vi "梦幻城堡C1~3通信.vi"() -> ()   [LabVIEW 2016, in "环境动力监测库.lvlib" / "UPS库.lvlib"]
uses:
  <vilib>/Instr/_visa.llb/VISA Configure Serial Port (Instr).vi
panel:
  out "Status":T1
  in  "open":bool
  in  "close":bool
  out "通信指示":bool
  in  "关机":bool
  in  "状态查询":bool
  out "读取缓冲区":string
  # "输入电压"
  # "输入故障电压"
  # "输出电压"
  # "输出电流百分比"
  # "输入频率"
  # "电池电压"
  # "UPS温度"
  # "UPS状态"
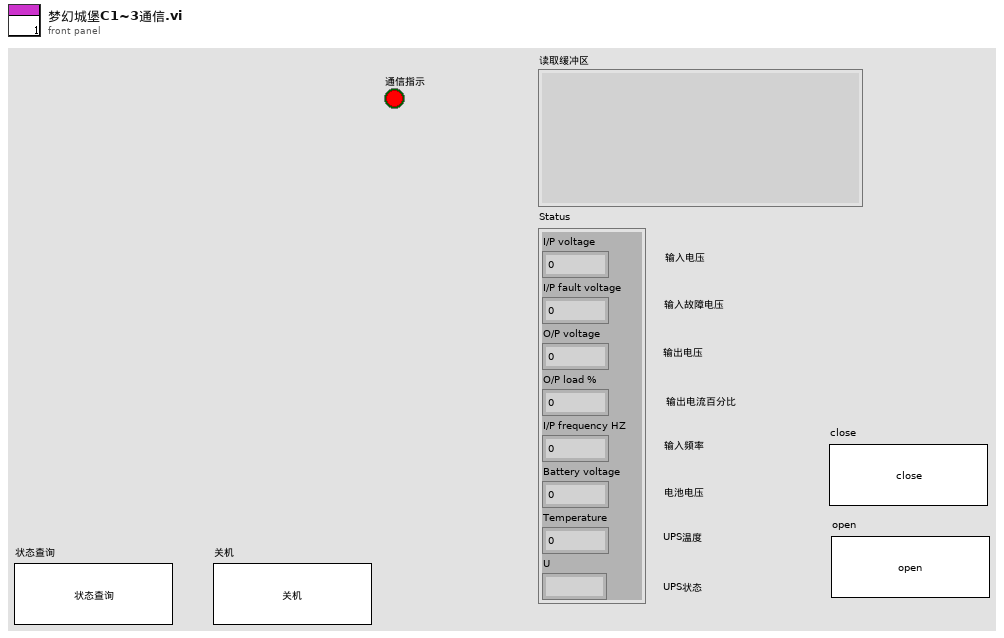
[diagram p1: front panel]
types:
  T1 = cluster{"I/P voltage":dbl, "I/P fault voltage":dbl, "O/P voltage":dbl, "O/P load %":dbl, "I/P frequency HZ":dbl, "Battery voltage":dbl, "Temperature":dbl, "U":string}
  T2 = cluster{"枚举":enum16{"open", "read", "write", "close"}, "写入缓冲区":string}
  T3 = typedef "环境动力监测库.lvlib/UPS库.lvlib/UPS型号.ctl" = enum16{"山特UPSC1~3", "山特UPSC6~20", "华为UPS2000-G-(1-3KVA)", "Kstar"}
  T4 = cluster{"VISA resource name":refnum<visa-resource-name>, "Serial Config":cluster{"baud rate (9600)":u32, "stop bits (10: 1 bit)":u16, "parity (0:none)":enum16{"None", "Odd", "Even", "Mark", "Space"}, "data bits (8)":u16, "timeout (10sec)":u32}, "型号选择":T3, "HW-UPS-2000 MB session":refnum<class "MB_Master.lvclass">, "连接方式":enum16{"串口", "TCP"}, "IP":string, "Port":string, "低电量报警阈值":u16, "功能启用":bool}
  T5 = cluster{"baud rate (9600)":u32, "stop bits (10: 1 bit)":u16, "parity (0:none)":enum16{"None", "Odd", "Even", "Mark", "Space"}, "data bits (8)":u16, "timeout (10sec)":u32}
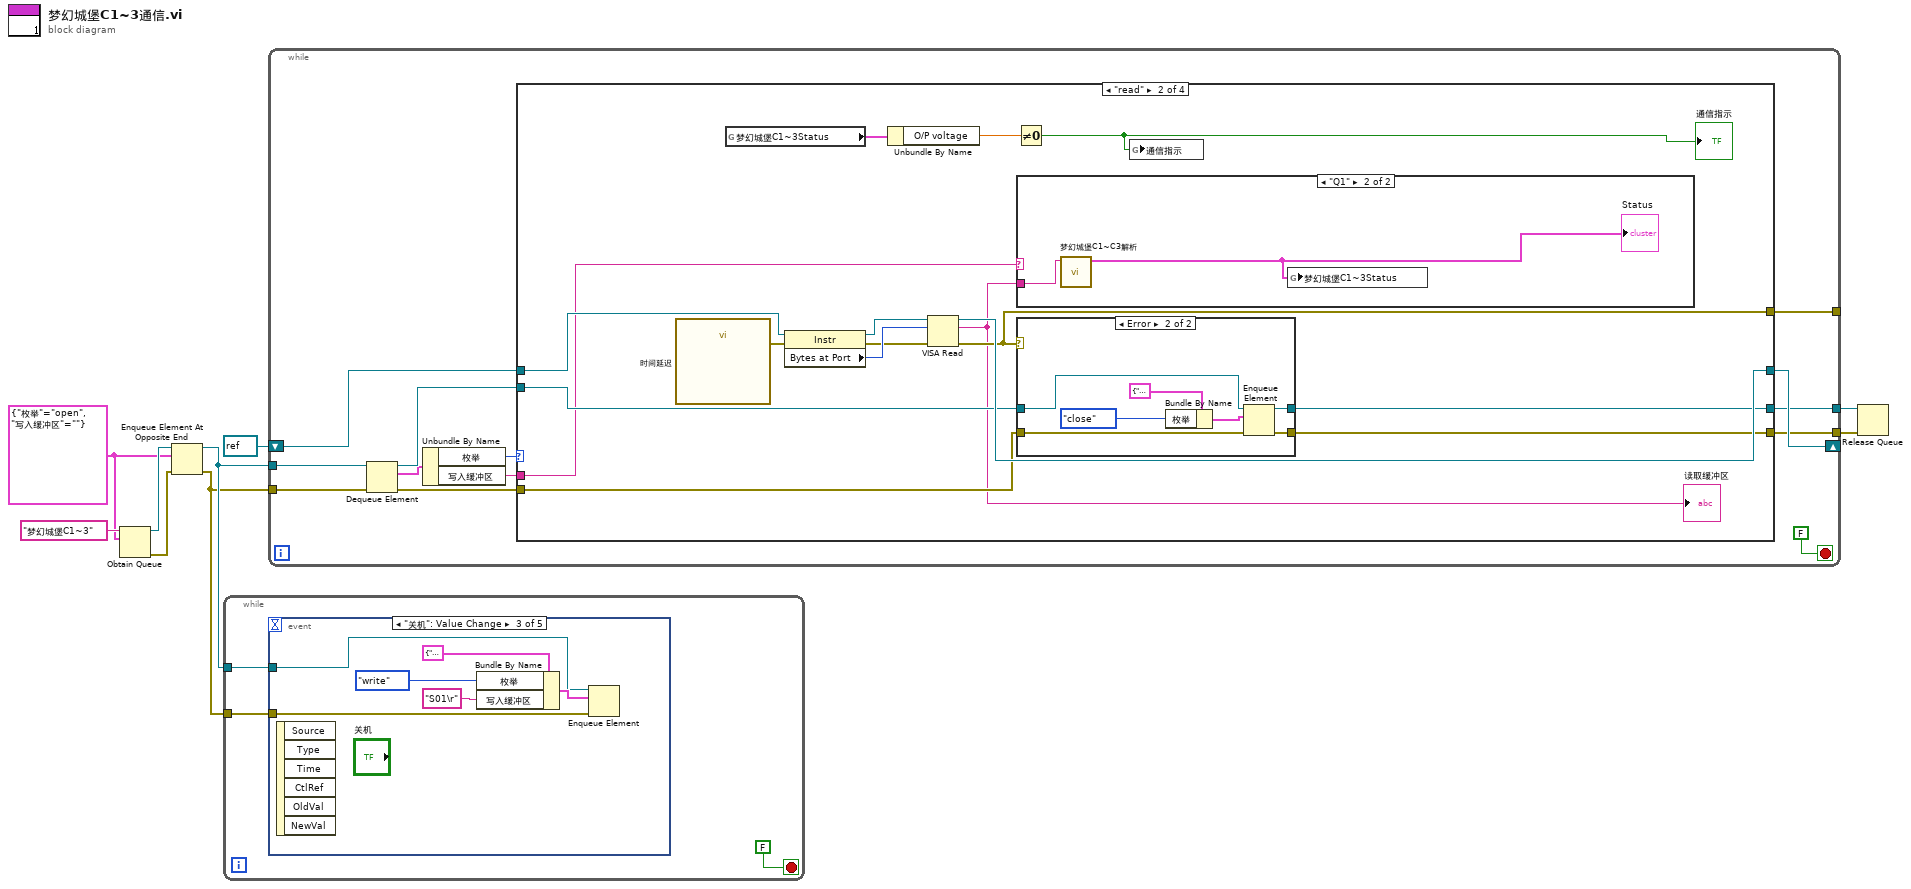
[diagram p0: block diagram]
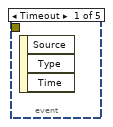
[diagram p2: hidden frame]
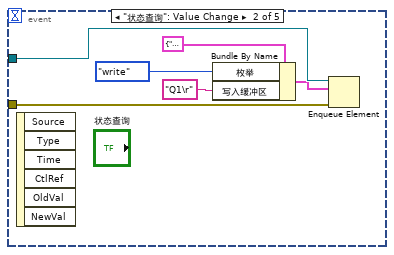
[diagram p3: hidden frame]
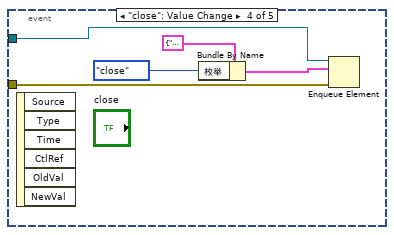
[diagram p4: hidden frame]
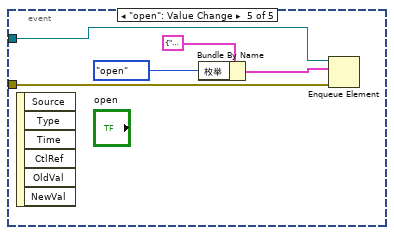
[diagram p5: hidden frame]
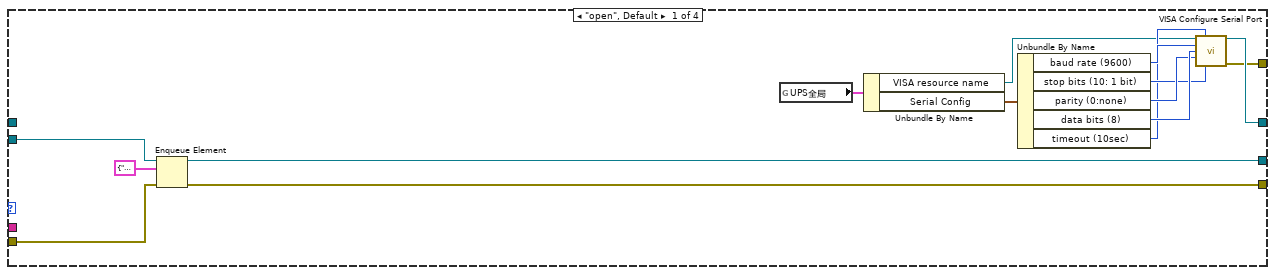
[diagram p6: hidden frame]
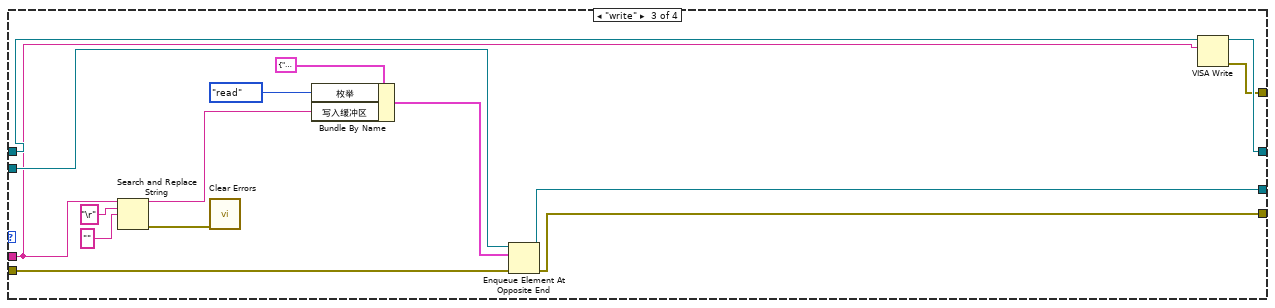
[diagram p9: hidden frame]
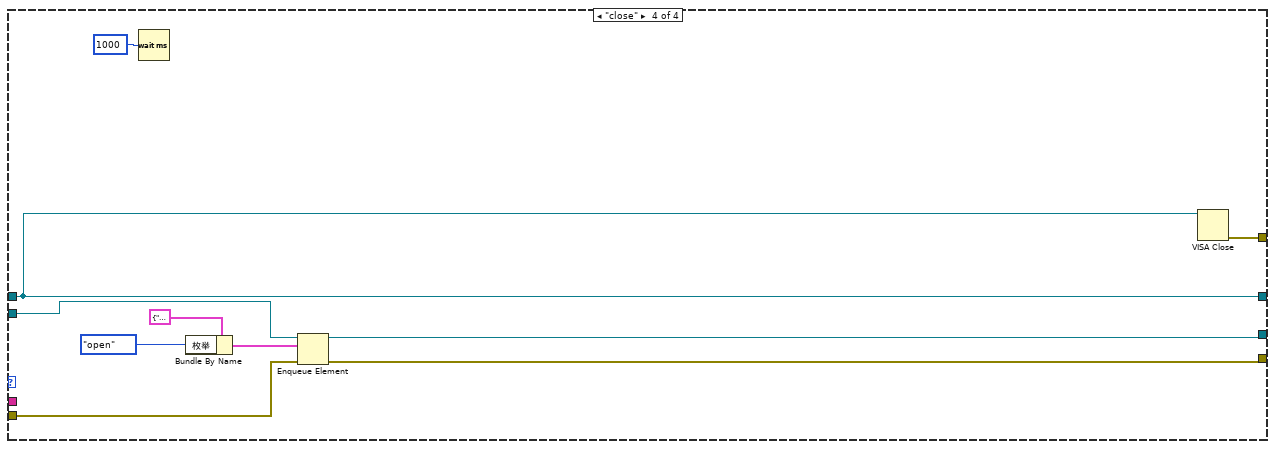
[diagram p10: hidden frame]
diagram:
  w3 = T2 {"枚举"=enum."open", "写入缓冲区"=""}
  n1 = Obtain Queue(name (unnamed)="梦幻城堡C1~3" ("名称（未命名）"), element data type=w3) -> (queue out=w8:refnum<queue>, error out=w7:errorcluster)  [unwired: 3 in, 1 out]
  n2 = Enqueue Element At Opposite End(queue=w8, element=w3, error in (no error)=w7) -> (queue out=w6:refnum<queue>, error out=w5:errorcluster)  [unwired: 1 in, 1 out]
  n3 = while {
    tunnel: w6 -> [w11]
    tunnel: w5 -> [w10]
    stop <- FALSE stop-if-true
    n4 = event shown="[2] \"关机\": Value Change" {
      selector: _ -> [_ _ _ _ _]
      dyn-events: _ -> [_ _ _ _ _]
      timeout: _ -> [_ _ _ _ _]
      tunnel: w11 -> [_ w17 w21 w29 w34]
      tunnel: w10 -> [_ w13 w20 w28 w33]
      event Timeout {
        n5 = event-data() -> ()  [unwired: 1 in, 3 out]
      }
      event "状态查询": Value Change {
        n6 = event-data() -> ()  [unwired: 1 in, 6 out]
        n7 = Bundle By Name(cluster=T2 {"枚举"=enum."open", "写入缓冲区"=""}, "枚举"=enum16{"open", "read", "write", "close"}."write" ("元素"), "写入缓冲区"="Q1\r") -> (w16:T2)
        n8 = Enqueue Element(queue=w17, element=w16, error in (no error)=w13) -> ()  [unwired: 1 in, 3 out]
      }
      event "关机": Value Change {
        n9 = event-data() -> ()  [unwired: 1 in, 6 out]
        n10 = Bundle By Name(cluster=T2 {"枚举"=enum."open", "写入缓冲区"=""}, "枚举"=enum16{"open", "read", "write", "close"}."write" ("元素"), "写入缓冲区"="S01\r") -> (w23:T2)
        n11 = Enqueue Element(queue=w21, element=w23, error in (no error)=w20) -> ()  [unwired: 1 in, 3 out]
      }
      event "close": Value Change {
        n12 = event-data() -> ()  [unwired: 1 in, 6 out]
        n13 = Bundle By Name(cluster=T2 {"枚举"=enum."open", "写入缓冲区"=""}, "枚举"=enum16{"open", "read", "write", "close"}."close") -> (w25:T2)
        n14 = Enqueue Element(queue=w29, element=w25, error in (no error)=w28) -> ()  [unwired: 1 in, 3 out]
      }
      event "open": Value Change {
        n15 = event-data() -> ()  [unwired: 1 in, 6 out]
        n16 = Bundle By Name(cluster=T2 {"枚举"=enum."open", "写入缓冲区"=""}, "枚举"=enum16{"open", "read", "write", "close"}."open") -> (w30:T2)
        n17 = Enqueue Element(queue=w34, element=w30, error in (no error)=w33) -> ()  [unwired: 1 in, 3 out]
      }
    }
  }
  n18 = while {
    shift-right: [w47] -> _
    shift-left: refnum<visa-resource-name> refnum ("VISA resource name out") -> [w46]
    tunnel: [w45] -> _
    tunnel: w6 -> [w43]
    tunnel: w5 -> [w42]
    tunnel: [w38] -> w1
    tunnel: [w39] -> w2
    stop <- FALSE stop-if-true
    n19 = Dequeue Element(queue=w43, error in (no error)=w42) -> (queue out=w41:refnum<queue>, element=w37:T2, error out=w40:errorcluster)  [unwired: 1 in, 1 out]
    n20 = Unbundle By Name(w37) -> ("枚举"=w36:enum16{"open", "read", "write", "close"}, "写入缓冲区"=w35:string)
    n21 = case shown="\"read\"" w36 {
      tunnel: [w62 w75 w103 w113] -> w47
      tunnel: w46 -> [_ w78 w104 w113]
      tunnel: [w61 w73 w102 w114] -> w45
      tunnel: w41 -> [w55 w72 w101 w109]
      tunnel: w40 -> [w54 w71 w100 w108]
      tunnel: [w53 w70 w96 w107] -> w39
      tunnel: [w52 w69 w95 w106] -> w38
      tunnel: w35 -> [_ w68 w94 _]
      frame "open", Default {
        n22 = Enqueue Element(queue=w55, element=T2 {"枚举"=enum."read", "写入缓冲区"=""}, error in (no error)=w54) -> (queue out=w53:refnum<queue>, error out=w52:errorcluster)  [unwired: 1 in, 1 out]
        n23 = global read "断电保存全局变量.vi" "UPS全局"() -> (w50:T4)
        n24 = Unbundle By Name(w50) -> ("VISA resource name"=w48:refnum<visa-resource-name>, "Serial Config"=w49:T5)
        n25 = Unbundle By Name(w49) -> ("baud rate (9600)"=w60:u32, "stop bits (10: 1 bit)"=w57:u16, "parity (0:none)"=w58:enum16{"None", "Odd", "Even", "Mark", "Space"}, "data bits (8)"=w59:u16, "timeout (10sec)"=w56:u32)
        n26 = call-poly "VISA Configure Serial Port"("VISA resource name"=w48, "timeout (10sec)"=w56, "baud rate (9600)"=w60, "data bits (8)"=w59, "parity (0:none)"=w58, "stop bits (10: 1 bit)"=w57) -> ("VISA resource name out"=w62:refnum<visa-resource-name>, "error out"=w61:errorcluster)  [unwired: 8 in]
      }
      frame "read" {
        n27 = call "时间延迟"() -> ("error out"=w74:errorcluster)  [unwired: 11 in]
        n28 = global read "UPS内部交互全局.vi" "梦幻城堡C1~3Status"() -> (w65:T1)
        n29 = property class="Instr"(reference=w78, error in=w74) -> (reference out=w76:refnum<visa-resource-name>, error out=w67:errorcluster, "Bytes at Port"=w77:u32)
        n30 = Unbundle By Name(w65) -> ("O/P voltage"=w64:dbl)
        n31 = VISA Read(VISA resource name=w76, byte count=w77, error in (no error)=w67) -> (VISA resource name out=w75:refnum<visa-resource-name>, read buffer=w66:string, error out=w73:errorcluster)  [unwired: 1 out]
        "读取缓冲区" <- w66
        n32 = Not Equal To 0?(x=w64) -> (x != 0?=w63:bool)
        "通信指示" <- w63
        n33 = case shown="\"Q1\"" w68 {
          tunnel: w66 -> [_ w79]
          frame "假", Default {
          }
          frame "Q1" {
            n34 = call "梦幻城堡C1~C3解析.vi"("读取缓冲区"=w79) -> ("Status"=w80:T1)  [unwired: 10 in]
            "Status" <- w80
            n35 = global write "UPS内部交互全局.vi" "梦幻城堡C1~3Status"(w80) -> ()
          }
        }
        n36 = case shown="Error" w73 {
          tunnel: w72 -> [w82 w83]
          tunnel: w71 -> [w81 w86]
          tunnel: [w82 w85] -> w70
          tunnel: [w81 w84] -> w69
          frame No Error {
          }
          frame Error {
            n37 = Bundle By Name(cluster=T2 {"枚举"=enum."open", "写入缓冲区"=""}, "枚举"=enum16{"open", "read", "write", "close"}."close") -> (w88:T2)
            n38 = Enqueue Element(queue=w83, element=w88, error in (no error)=w86) -> (queue out=w85:refnum<queue>, error out=w84:errorcluster)  [unwired: 1 in, 1 out]
          }
        }
        n39 = global write "UPS内部交互全局.vi" "通信指示"(w63) -> ()
      }
      frame "write" {
        n40 = Search and Replace String(input string=w94, search string="\r" ("搜索字符串"), replace string="" ("替换字符串(\"\")")) -> (result string=w91:string, error out=w90:errorcluster)  [unwired: 5 in, 2 out]
        n41 = call <vilib>:"Clear Errors.vi"("error in (no error)"=w90) -> ()  [unwired: 5 in, 2 out]
        n42 = Bundle By Name(cluster=T2 {"枚举"=enum."open", "写入缓冲区"=""}, "枚举"=enum16{"open", "read", "write", "close"}."read", "写入缓冲区"=w91) -> (w97:T2)
        n43 = Enqueue Element At Opposite End(queue=w101, element=w97, error in (no error)=w100) -> (queue out=w96:refnum<queue>, error out=w95:errorcluster)  [unwired: 1 in, 1 out]
        n44 = VISA Write(VISA resource name=w104, write buffer=w94) -> (VISA resource name out=w103:refnum<visa-resource-name>, error out=w102:errorcluster)  [unwired: 1 in, 1 out]
      }
      frame "close" {
        n45 = Wait (ms)(milliseconds to wait=u32 1000 ("等待时间（毫秒）")) -> ()  [unwired: 1 out]
        n46 = Bundle By Name(cluster=T2 {"枚举"=enum."open", "写入缓冲区"=""}, "枚举"=enum16{"open", "read", "write", "close"}."open") -> (w110:T2)
        n47 = Enqueue Element(queue=w109, element=w110, error in (no error)=w108) -> (queue out=w107:refnum<queue>, error out=w106:errorcluster)  [unwired: 1 in, 1 out]
        n48 = VISA Close(VISA resource name=w113) -> (error out=w114:errorcluster)  [unwired: 1 in]
      }
    }
  }
  n49 = Release Queue(queue=w2, error in (no error)=w1) -> ()  [unwired: 1 in, 3 out]
